vi "SetZElevAper_modify.vi"(6 "Mode":string(combo)="DProbe", 7 "focusRangeCm":sgl format="%.2f", 8 "error in (no error)":errorcluster, 9 "timeout (ms)":i32=40000, 10 "elevAperIndex":i8, 11 "connection ID in":refnum<k5>) -> (0 "error out":errorcluster, 1 "SwitchDepth":sgl[](array[numeric]), 2 "probeNumElevAper":i32, 3 "connection ID out":refnum<k5>)   [LabVIEW 2016]
doc: "Sets the Z system elevation aperture to the value specified by elevAperIndex (0 for one row active, 1 for three rows active, etc.). It first reads the number of possible values of this index (1 or 2 for a one or three row transducer, respectively):\n Imaging Control Layer.\n ProbeRootPc.\n CommonProbe.\n ProbeNumElevAper\nNext, it reads the current switch depth array:\n Imaging Control Layer.\n ProbeRootPc.\n DProbe.\n ElevAperSwitchDepthCmA\nand compares it with the input focusRangeCm. If rows are to be active, the switch depth should be less than the focus; otherwise it should be greater. If the switch depth is on the wrong side of the focus, the program sets it to either 0 or focus+1 to give the correct elevation aperture. For a one row probe, no action is taken after reading NumElevAper."
panel:
  out "Pre_SwitchDepth":sgl[](array[numeric])
  # "Program constants"
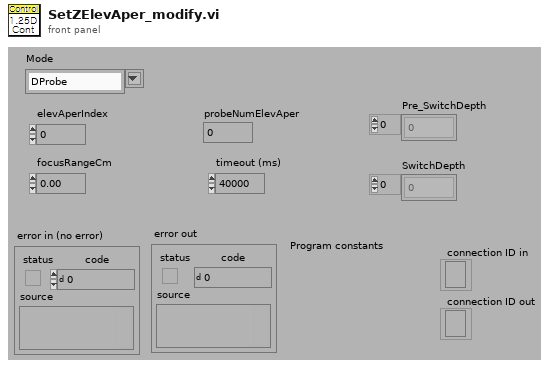
[diagram p1: front panel]
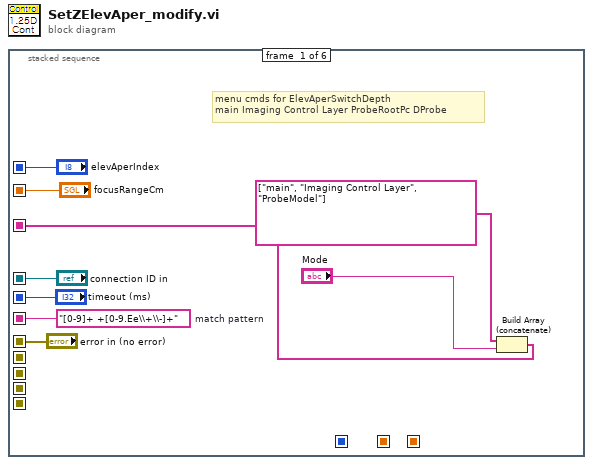
[diagram p0: block diagram]
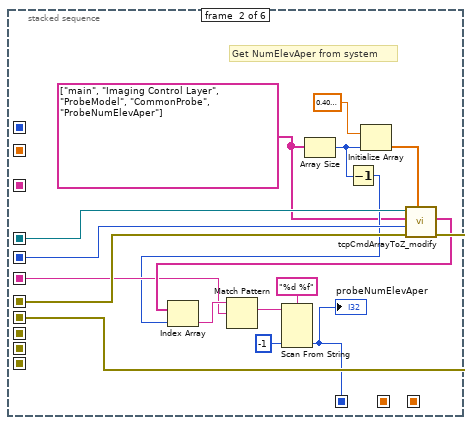
[diagram p2: hidden frame]
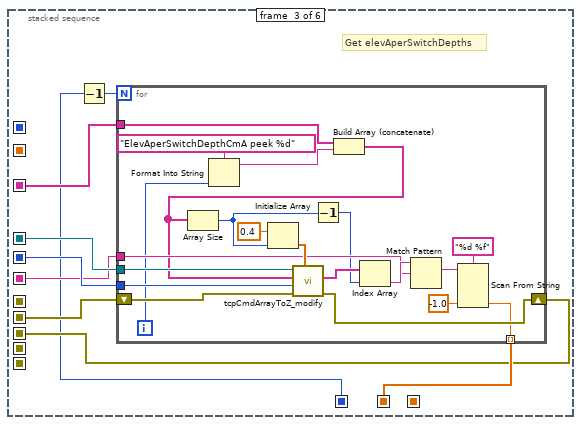
[diagram p3: hidden frame]
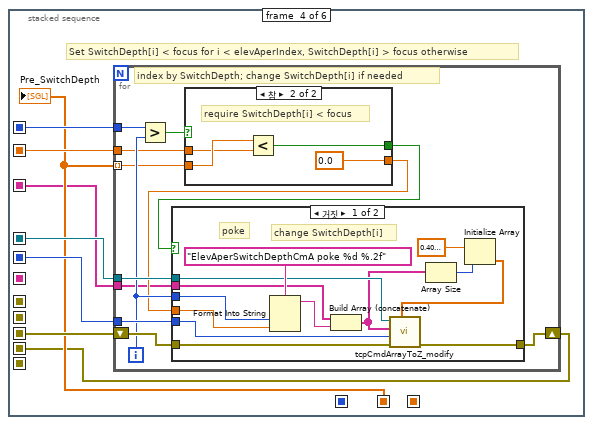
[diagram p4: hidden frame]
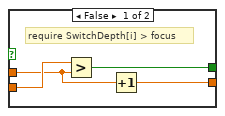
[diagram p6: hidden frame]
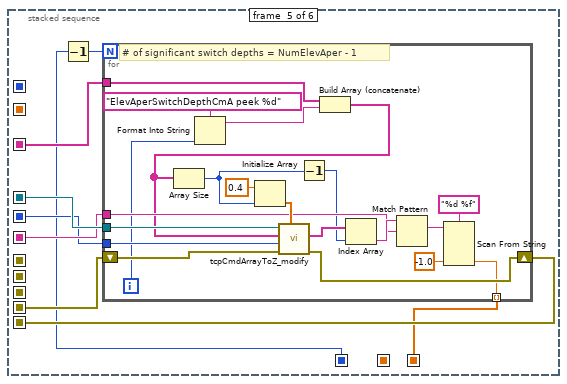
[diagram p7: hidden frame]
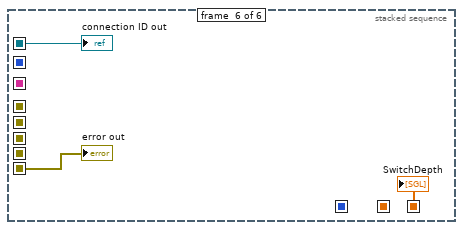
[diagram p8: hidden frame]
diagram:
  n1 = stacked-sequence {
    seq-local: ["error in (no error)" _ _ _ _ _] -> [_ w21 _ _ _ _]
    seq-local: ["timeout (ms)" _ _ _ _ _] -> [_ w22 w33 w61 w100 _]
    seq-local: ["elevAperIndex" _ _ _ _ _] -> [_ _ _ w59 _ _]
    seq-local: ["connection ID in" _ _ _ _ _] -> [_ w23 w34 w62 w102 w128]
    seq-local: [_ w20 _ _ _ _] -> [_ _ w32 _ _ _]
    seq-local: [w5 _ _ _ _ _] -> [_ w15 w31 _ w101 _]
    seq-local: [_ w10 _ _ _ _] -> [_ _ w27 _ w98 _]
    seq-local: [_ _ w30 _ _ _] -> [_ _ _ w57 _ _]
    seq-local: [_ _ w29 _ _ _] -> [_ _ _ w60 _ _]
    seq-local: ["focusRangeCm" _ _ _ _ _] -> [_ _ _ w58 _ _]
    seq-local: [_ _ _ w56 _ _] -> [_ _ _ _ w105 _]
    seq-local: [w2 _ _ _ _ _] -> [_ _ w28 w55 w103 _]
    seq-local: [_ _ _ _ w104 _] -> [_ _ _ _ _ w127]
    seq-local: [_ _ _ _ w99 _] -> [_ _ _ _ _ w126]
    frame #0 {
      w5 = "[0-9]+ +[0-9.Ee\\+\\-]+"  # match pattern
      # "menu cmds for ElevAperSwitchDepth\nmain Imaging Control Layer ProbeRootPc DProbe"
      n2 = Build Array (concatenate)(string[] ["main", "Imaging Control Layer", "ProbeModel"] ("menu cmds for NumElevAper\nmain Imaging Control Layer ProbeRootPc CommonProbe"), "Mode") -> (w2:string[])
    }
    frame #1 {
      w12 = string[] ["main", "Imaging Control Layer", "ProbeModel", "CommonProbe", "ProbeNumElevAper"] ("menu cmds for NumElevAper\nmain Imaging Control Layer ProbeRootPc CommonProbe")
      # "Get NumElevAper from system"
      n3 = Array Size(array=w12) -> (size(s)=w13:i32)
      n4 = Decrement(x=w13) -> (x-1=w14:i32)
      n5 = Initialize Array(sgl 0.4 ("Element Data"), w13) -> (w24:sgl[])
      n6 = call "tcpCmdArrayToZ_modify.vi"("Delay (sec)"=w24, "error in (no error)"=w21, "Timeout (ms)"=w22, "Command array"=w12, "connection ID in"=w23) -> ("error out"=w20:errorcluster, "Receive array"=w17:string[])  [unwired: 2 in, 3 out]
      n7 = Index Array(array=w17, index=w14) -> (element=w16:string)
      n8 = Match Pattern(string=w16, regular expression=w15) -> (match substring=w19:string)  [unwired: 1 in, 3 out]
      n9 = Scan From String(format string="%d %f" ("Format String"), input string=w19, default 2=-1 ("Default Value 2")) -> (output 2=w10:i32)  [unwired: 4 in, 3 out]
      "probeNumElevAper" <- w10
    }
    frame #2 {
      # "Get elevAperSwitchDepths"
      n10 = Decrement(x=w27) -> (x-1=w26:i32)
      n11 = for {
        N: w26 -> [_]
        tunnel: w34 -> [w53]
        tunnel: w33 -> [w52]
        shift-right: [w47] -> w29
        shift-left: w32 -> [w51]
        tunnel: w31 -> [w45]
        tunnel: [w36] -> w30 mode=indexing
        tunnel: w28 -> [w41]
        i -> [w42]
        n12 = Format Into String(format string="ElevAperSwitchDepthCmA peek %d" ("Format String"), w42) -> (resulting string=w38:string)  [unwired: 2 in, 1 out]
        n13 = Build Array (concatenate)(w41, w38) -> (w40:string[])
        n14 = Array Size(array=w40) -> (size(s)=w44:i32)
        n15 = Initialize Array(0.4, w44) -> (w54:dbl[])
        n16 = call "tcpCmdArrayToZ_modify.vi"("Delay (sec)"=w54, "error in (no error)"=w51, "Timeout (ms)"=w52, "Command array"=w40, "connection ID in"=w53) -> ("error out"=w47:errorcluster, "Receive array"=w46:string[])  [unwired: 2 in, 3 out]
        n17 = Decrement(x=w44) -> (x-1=w43:i32)
        n18 = Index Array(array=w46, index=w43) -> (element=w48:string)
        n19 = Match Pattern(string=w48, regular expression=w45) -> (match substring=w50:string)  [unwired: 1 in, 3 out]
        n20 = Scan From String(format string="%d %f" ("Format String"), input string=w50, default 2=sgl -1.0 ("Default Value 2")) -> (output 2=w36:sgl)  [unwired: 4 in, 3 out]
      }
    }
    frame #3 {
      # "Set SwitchDepth[i] < focus for i < elevAperIndex, SwitchDepth[i] > focus otherwise"
      n21 = for {
        tunnel: w62 -> [w74]
        tunnel: w61 -> [w73]
        shift-right: [w71] -> w56
        shift-left: w60 -> [w72]
        tunnel: w59 -> [w70]
        tunnel: w58 -> [w66]
        tunnel: w57 -> [w67] mode=indexing
        tunnel: w55 -> [w63]
        i -> [w69]
        # "index by SwitchDepth; change SwitchDepth[i] if needed"
        n22 = Greater?(x=w70, y=w69) -> (0:w68:bool)
        n23 = case shown="참" w68 {
          tunnel: w67 -> [w92 w96]
          tunnel: w66 -> [w90 w95]
          tunnel: [w91 w94] -> w65
          tunnel: [w89 sgl 0.0] -> w64
          frame False {
            # "require SwitchDepth[i] > focus"
            n24 = Greater?(x=w92, y=w90) -> (0:w91:bool)
            n25 = Increment(x=w90) -> (x+1=w89:sgl)
          }
          frame True {
            # "require SwitchDepth[i] < focus"
            n26 = Less?(x=w96, y=w95) -> (x < y?=w94:bool)
          }
        }
        n27 = case shown="거짓" w65 {
          tunnel: w74 -> [w85 _]
          tunnel: w73 -> [w84 _]
          tunnel: w72 -> [w83 w88]
          tunnel: [w82 w88] -> w71
          tunnel: w69 -> [w81 _]
          tunnel: w64 -> [w80 _]
          tunnel: w63 -> [w79 _]
          frame False {
            # "poke"
            # "change SwitchDepth[i]"
            n28 = Format Into String(format string="ElevAperSwitchDepthCmA poke %d %.2f", w81, w80) -> (resulting string=w86:string)  [unwired: 2 in, 1 out]
            n29 = Build Array (concatenate)(w79, w86) -> (w77:string[])
            n30 = Array Size(array=w77) -> (size(s)=w76:i32)
            n31 = Initialize Array(sgl 0.4 ("Element Data"), w76) -> (w75:sgl[])
            n32 = call "tcpCmdArrayToZ_modify.vi"("Delay (sec)"=w75, "error in (no error)"=w83, "Timeout (ms)"=w84, "Command array"=w77, "connection ID in"=w85) -> ("error out"=w82:errorcluster)  [unwired: 2 in, 4 out]
          }
          frame True {
            # "SwitchDepth[i] is ok; no change"
          }
        }
      }
      "Pre_SwitchDepth" <- w57
    }
    frame #4 {
      n33 = Decrement(x=w98) -> (x-1=w97:i32)
      n34 = for {
        N: w97 -> [_]
        tunnel: w102 -> [w124]
        tunnel: w100 -> [w123]
        shift-right: [w118] -> w104
        shift-left: w105 -> [w122]
        tunnel: w101 -> [w116]
        tunnel: [w107] -> w99 mode=indexing
        tunnel: w103 -> [w112]
        i -> [w113]
        # "# of significant switch depths = NumElevAper - 1"
        n35 = Format Into String(format string="ElevAperSwitchDepthCmA peek %d" ("Format String"), w113) -> (resulting string=w109:string)  [unwired: 2 in, 1 out]
        n36 = Build Array (concatenate)(w112, w109) -> (w111:string[])
        n37 = Array Size(array=w111) -> (size(s)=w115:i32)
        n38 = Initialize Array(0.4, w115) -> (w125:dbl[])
        n39 = call "tcpCmdArrayToZ_modify.vi"("Delay (sec)"=w125, "error in (no error)"=w122, "Timeout (ms)"=w123, "Command array"=w111, "connection ID in"=w124) -> ("error out"=w118:errorcluster, "Receive array"=w117:string[])  [unwired: 2 in, 3 out]
        n40 = Decrement(x=w115) -> (x-1=w114:i32)
        n41 = Index Array(array=w117, index=w114) -> (element=w119:string)
        n42 = Match Pattern(string=w119, regular expression=w116) -> (match substring=w121:string)  [unwired: 1 in, 3 out]
        n43 = Scan From String(format string="%d %f" ("Format String"), input string=w121, default 2=sgl -1.0 ("Default Value 2")) -> (output 2=w107:sgl)  [unwired: 4 in, 3 out]
      }
    }
    frame #5 {
      "error out" <- w127
      "connection ID out" <- w128
      "SwitchDepth" <- w126
    }
  }
